vi "checkauto.vi"(0 "G-Code Array":string[](array[string]), 2 "Start Auto":bool, 3 "error in (no error)":errorcluster, 4 "queue":T1) -> (10 "error out":errorcluster)   [LabVIEW 2017, in "LibraryGcode.lvlib"]
uses:
  LibraryGcode.lvlib
  control/Queue/QueueCMDandPOS.ctl
  control/Queue/TypeDataPOS.ctl
  control/stateCmdUpdatePara.ctl
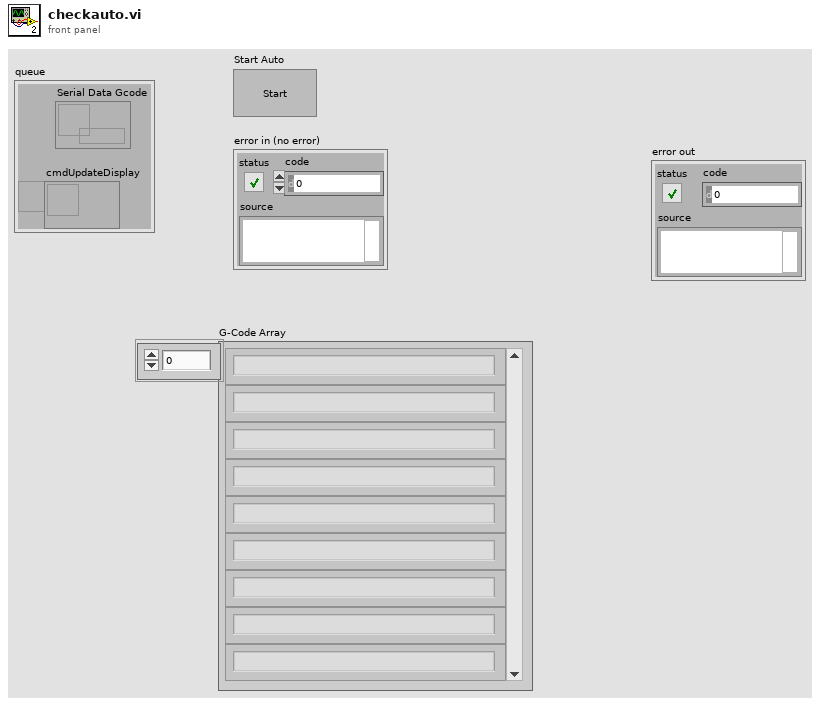
[diagram p1: front panel]
types:
  T1 = typedef "LibraryGcode.lvlib/QueueCMDandPOS.ctl" = cluster{"Serial Data Gcode":refnum<queue>, "cmdUpdateDisplay":refnum<queue>}
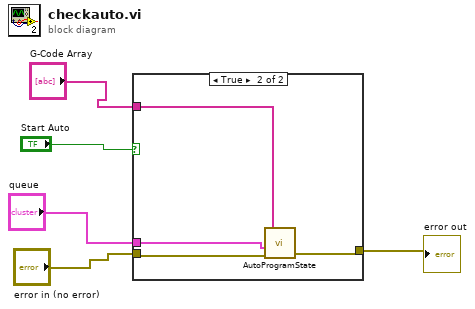
[diagram p0: block diagram]
diagram:
  n1 = case shown="True" "Start Auto" {
    tunnel: "error in (no error)" -> [w6 w7]
    tunnel: "queue" -> [_ w10]
    tunnel: [w6 w8] -> w2
    tunnel: "G-Code Array" -> [_ w9]
    frame False {
    }
    frame True {
      n2 = call "AutoProgramState.vi"("error in (no error)"=w7, "INcluster"=w10, "G-Code Array"=w9) -> ("error in (no error) 2"=w8:errorcluster)  [unwired: 1 in, 2 out]
    }
  }
  "error out" <- w2
